vi "Run_Y_Train.vi"(8 "error in (no error)":errorcluster caption="entrée d'erreur (pas d'erreur)", 9 "Y":string[][](array[string]), 10 "X":string[][](array[string]), 11 "TrainTest.lvclass":refnum<class "TrainTest.lvclass">) -> (0 "error out":errorcluster caption="sortie d'erreur", 2 "Data":T1, 3 "TrainTest.lvclass":refnum<class "TrainTest.lvclass">)   [LabVIEW 2020, in "TrainTest.lvclass"]
doc: "Returns : \n\n- splitting : list, \n List containing Y_TRAIN"
uses:
  TrainTest.lvclass
  TrainTest.lvclass/TrainTest.ctl
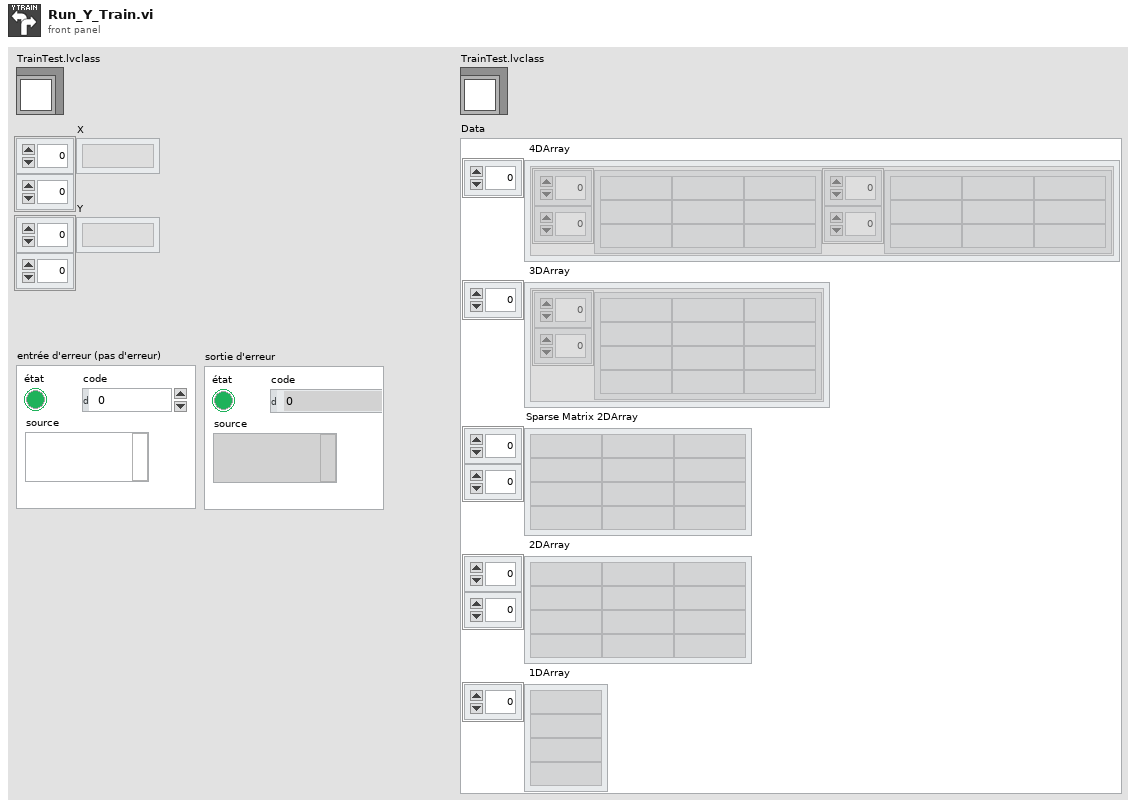
[diagram p1: front panel]
types:
  T1 = cluster{" 4DArray":cluster{"1":string[][], "2":string[][]}[], " 3DArray":cluster{"Tableau":string[][]}[], "Sparse Matrix 2DArray":string[][], " 2DArray":string[][], " 1DArray":string[]}
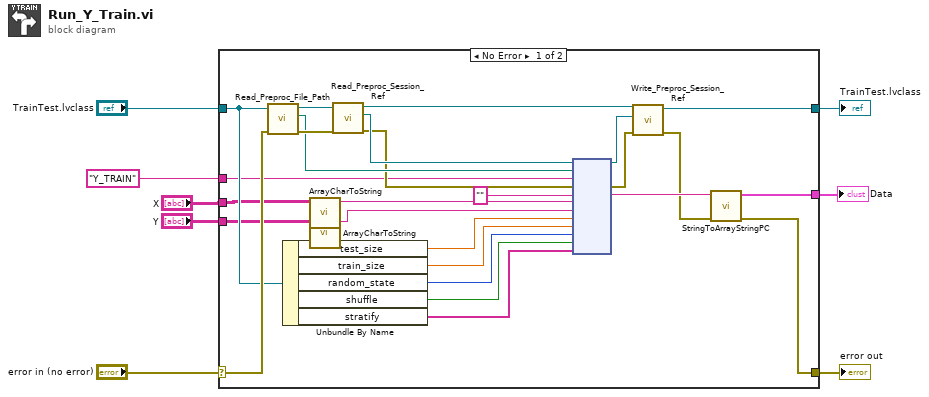
[diagram p0: block diagram]
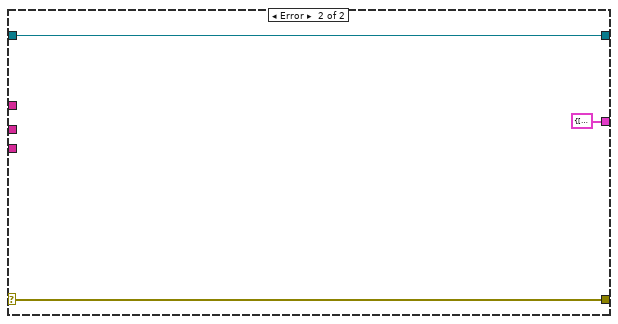
[diagram p2: hidden frame]
diagram:
  n1 = case shown="No Error" "error in (no error)" {
    selector: "error in (no error)" -> [w34 w37]
    tunnel: [w14 w37] -> w7
    tunnel: [w17 w36] -> w5
    tunnel: "TrainTest.lvclass" -> [w24 w36]
    tunnel: "Y_TRAIN" ("Fonction") -> [w23 _]
    tunnel: "X" -> [w12 _]
    tunnel: "Y" -> [w11 _]
    tunnel: [w13 T1 {" 4DArray"=[], " 3DArray"=[], "Sparse Matrix 2DArray"=[], " 2DArray"=[], " 1DArray"=[]} ("Data")] -> w1
    frame No Error {
      n2 = call-dynamic "Read_Preproc_File_Path.vi"("error in (no error)"=w34, "Python in"=w24) -> ("error out"=w32:errorcluster, "File_Path"=w31:path, "Python out"=w33:refnum<class "TrainTest.lvclass">)  [unwired: 7 in]
      n3 = Unbundle By Name(w24) -> ("test_size"=w22:dbl, "train_size"=w21:dbl, "random_state"=w20:i32, "shuffle"=w19:bool, "stratify"=w18:string[])
      n4 = call "ArrayCharToString.vi"("TAB"=w12) -> ("Instruction"=w10:string)  [unwired: 10 in]
      n5 = call "ArrayCharToString.vi"("TAB"=w11) -> ("Instruction"=w9:string)  [unwired: 10 in]
      n6 = call-dynamic "Read_Preproc_Session_Ref.vi"("error in (no error)"=w32, "Python in"=w33) -> ("error out"=w29:errorcluster, "Session_ref"=w30:refnum<k35>, "Python out"=w28:refnum<class "TrainTest.lvclass">)  [unwired: 7 in]
      n7 = node(w30, w31, w23, w29, "", w10, w9, w22, w21, w20, w19, w18) -> (w26:refnum<k35>, w27:errorcluster, w16:string)  [unwired: 7 in, 2 out]
      n8 = call-dynamic "Write_Preproc_Session_Ref.vi"("error in (no error)"=w27, "Session_ref"=w26, "Python in"=w28) -> ("error out"=w15:errorcluster, "Python out"=w17:refnum<class "TrainTest.lvclass">)  [unwired: 7 in]
      n9 = call "StringToArrayStringPC.vi"("sortie d'erreur"=w15, "Return value"=w16) -> ("sortie d'erreur"=w14:errorcluster, "Data"=w13:T1)  [unwired: 8 in]
    }
    frame Error {
    }
  }
  "error out" <- w7
  "TrainTest.lvclass" <- w5
  "Data" <- w1
